vi "Parse Float Data Array.vi"(8 "error in (no error)":errorcluster, 10 "Display":T1, 11 "Data Read":u8[][](array[numeric])) -> (0 "error out":errorcluster, 2 "output cluster":T1, 5 "Motor2RatingRPM":u16, 7 "Motor1RatingRPM":u16)   [LabVIEW 2018]
uses:
  Ctls/DisplayIndicator.ctl
  Ctls/MotroConfigData.ctl
  Ctls/MotorConfig.ctl
  Ctls/MagType.ctl
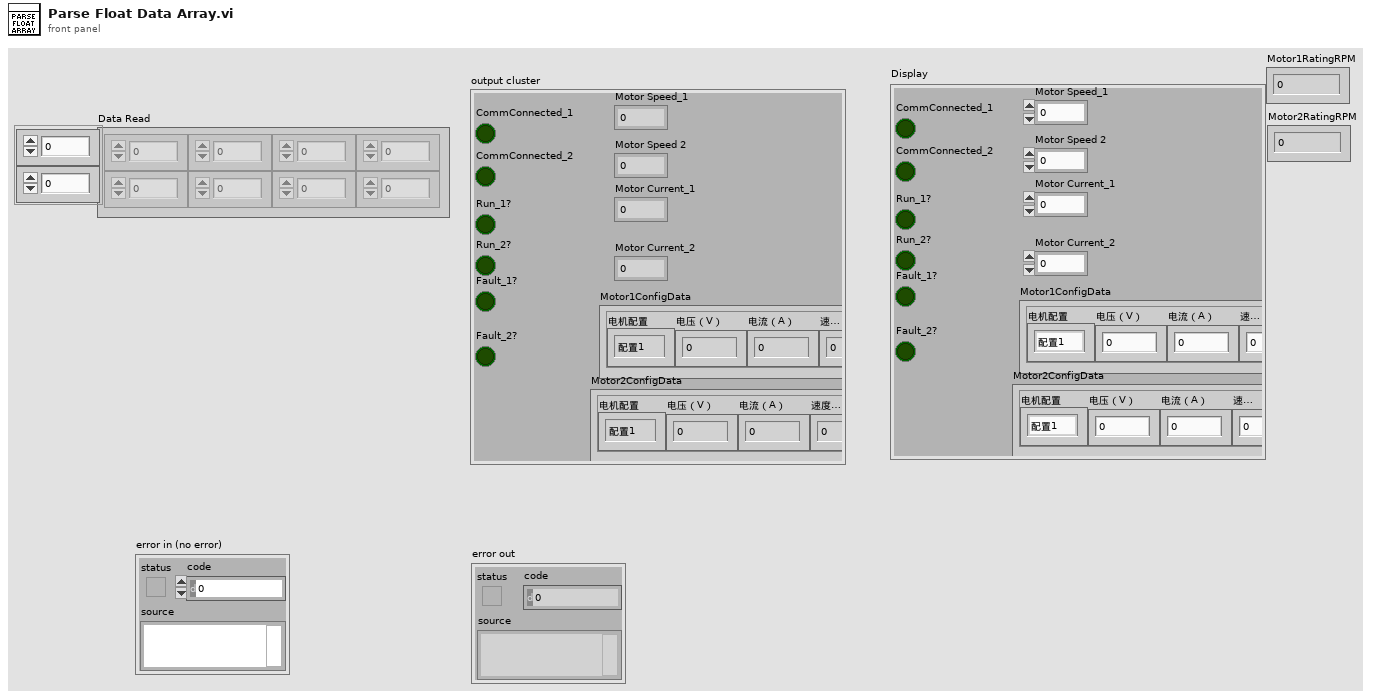
[diagram p1: front panel]
types:
  T1 = typedef "DisplayIndicator.ctl" = cluster{"CommConnected_1":bool, "Run_1?":bool, "Fault_1?":bool, "CommConnected_2":bool, "Run_2?":bool, "Fault_2?":bool, "Motor Speed 2":sgl, "Motor Speed_1":sgl, "Motor Current_1":sgl, "Motor Current_2":sgl, "Motor1ConfigData":T2, "Motor2ConfigData":T2}
  T2 = typedef "MotroConfigData.ctl" = cluster{"电机配置":T3, "电压（V）":dbl, "电流（A）":dbl, "速度（RPM）":dbl, "励磁方式":T4}
  T3 = typedef "MotorConfig.ctl" = enum16{"配置1", "配置2", "配置3", "配置4"}
  T4 = typedef "MagType.ctl" = enum16{"永磁", "励磁"}
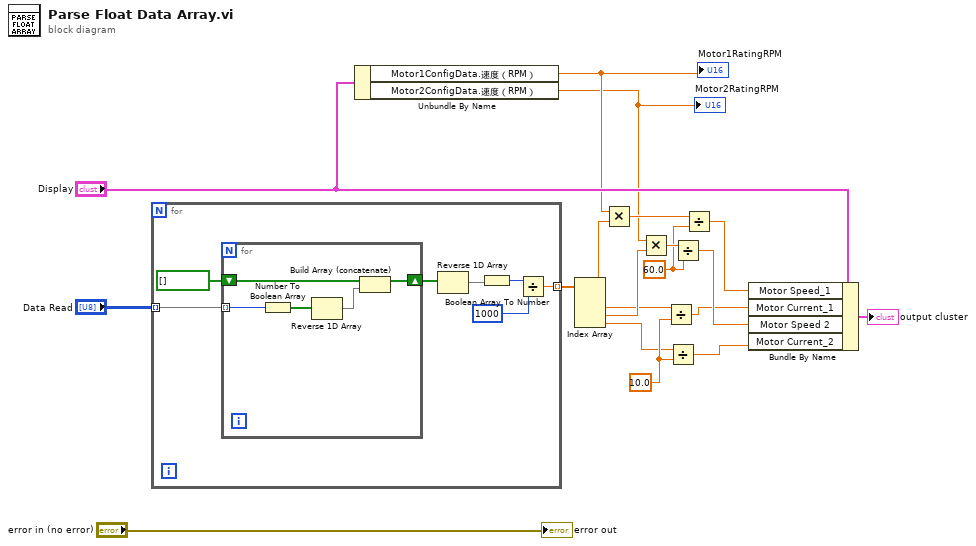
[diagram p0: block diagram]
diagram:
  w3 = 10.0 ("y")
  w11 = 60.0 ("y")
  n1 = for {
    tunnel: "Data Read" -> [w26] mode=indexing
    tunnel: [w20] -> w16 mode=indexing
    n2 = for {
      tunnel: w26 -> [w31] mode=indexing
      shift-right: [w29] -> w24
      shift-left: bool[] [] ("Boolean array") -> [w30]
      n3 = Number To Boolean Array(number=w31) -> (Boolean array=w28:bool[])
      n4 = Reverse 1D Array(array=w28) -> (reversed array=w27:bool[])
      n5 = Build Array (concatenate)(w30, w27) -> (w29:bool[])
    }
    n6 = Reverse 1D Array(array=w24) -> (reversed array=w23:bool[])
    n7 = Boolean Array To Number(Boolean array=w23) -> (number=w22:u32)
    n8 = Divide(x=w22, y=u16 1000) -> (x/y=w20:dbl)
  }
  n9 = Unbundle By Name("Display") -> ("Motor1ConfigData.速度（RPM）"=w7:dbl, "Motor2ConfigData.速度（RPM）"=w6:dbl)
  "Motor1RatingRPM" <- w7
  "Motor2RatingRPM" <- w6
  n10 = Index Array(array=w16) -> (element #1=w14:dbl, element #2=w5:dbl, element #3=w15:dbl, element #4=w2:dbl)  [unwired: 4 in]
  n11 = Multiply(x=w7, y=w14) -> (x*y=w12:dbl)
  n12 = Multiply(x=w6, y=w15) -> (x*y=w13:dbl)
  n13 = Divide(x=w5, y=w3) -> (x/y=w4:dbl)
  n14 = Divide(x=w2, y=w3) -> (x/y=w1:dbl)
  n15 = Divide(x=w13, y=w11) -> (x/y=w10:dbl)
  n16 = Divide(x=w12, y=w11) -> (x/y=w9:dbl)
  n17 = Bundle By Name(cluster="Display", "Motor Speed_1"=w9, "Motor Current_1"=w4, "Motor Speed 2"=w10, "Motor Current_2"=w1) -> (→"output cluster":T1)
  "error out" <- "error in (no error)"
